vi "Auto_Routine_DepositHighBackup.vi"   [LabVIEW 2020]
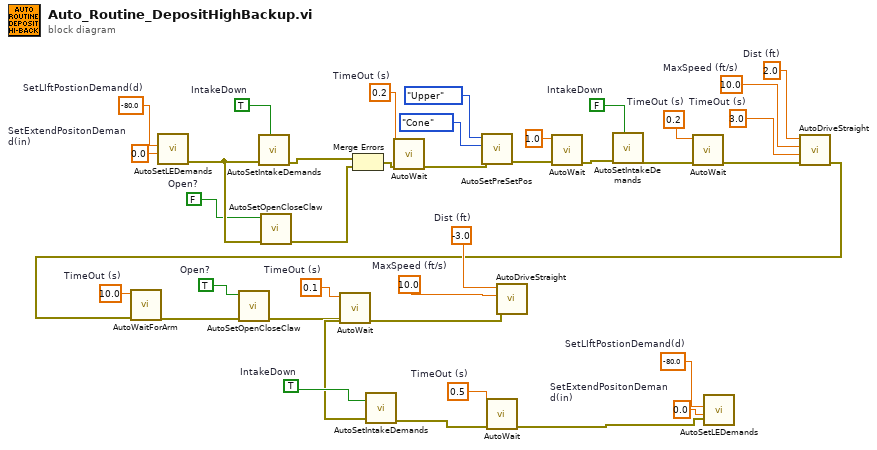
[diagram p0: block diagram]
diagram:
  w30 = 10.0  # MaxSpeed (ft/s)
  w26 = 3.0  # TimeOut (s)
  w25 = 10.0  # MaxSpeed (ft/s)
  w24 = 2.0  # Dist (ft)
  w23 = -80.0  # SetLIftPostionDemand(d)
  w22 = 0.0  # SetExtendPositonDemand(in)
  w21 = 0.5  # TimeOut (s)
  w20 = TRUE  # IntakeDown
  w18 = -3.0  # Dist (ft)
  w17 = 0.1  # TimeOut (s)
  w15 = TRUE  # Open?
  w13 = 0.2  # TimeOut (s)
  w12 = 10.0  # TimeOut (s)
  w7 = FALSE  # IntakeDown
  w5 = 0.2  # TimeOut (s)
  w4 = -80.0  # SetLIftPostionDemand(d)
  w3 = 0.0  # SetExtendPositonDemand(in)
  w2 = FALSE  # Open?
  w1 = TRUE  # IntakeDown
  n1 = call "AutoSetLEDemands.vi"("SetExtendPositonDemand(in)"=w3, "SetLIftPostionDemand(d)"=w4) -> ("error out"=w9:errorcluster)  [unwired: 9 in]
  n2 = call "AutoSetIntakeDemands.vi"("IntakeDown"=w1, "error in (no error)"=w9) -> ("error out"=w27:errorcluster)  [unwired: 9 in]
  n3 = call "AutoSetOpenCloseClaw.vi"("error in (no error)"=w9, "Open?"=w2) -> ("error out"=w28:errorcluster)  [unwired: 9 in]
  n4 = Merge Errors(w27, w28) -> (w29:errorcluster)
  n5 = call "AutoWait.vi"("error in (no error)"=w29, "TimeOut (s)"=w5) -> ("error out"=w6:errorcluster)  [unwired: 9 in]
  n6 = call "AutoSetPreSetPos.vi"("error in (no error)"=w6, "Game Piece"=enum16{"Cube", "Cone"}."Cone", "Position"=enum16{"Upper", "Lower", "Middle"}."Upper") -> ("error out"=w33:errorcluster)  [unwired: 8 in]
  n7 = call "AutoWait.vi"("error in (no error)"=w33, "TimeOut (s)"=1.0) -> ("error out"=w34:errorcluster)  [unwired: 9 in]
  n8 = call "AutoSetIntakeDemands.vi"("IntakeDown"=w7, "error in (no error)"=w34) -> ("error out"=w8:errorcluster)  [unwired: 9 in]
  n9 = call "AutoWait.vi"("error in (no error)"=w8, "TimeOut (s)"=w13) -> ("error out"=w10:errorcluster)  [unwired: 9 in]
  n10 = call "AutoDriveStraight.vi"("error in (no error)"=w10, "TimeOut (s)"=w26, "MaxSpeed (ft/s)"=w25, "Dist (ft)"=w24) -> ("error out"=w11:errorcluster)  [unwired: 7 in]
  n11 = call "AutoWaitForArm.vi"("error in (no error)"=w11, "TimeOut (s)"=w12) -> ("error out"=w14:errorcluster)  [unwired: 9 in]
  n12 = call "AutoSetOpenCloseClaw.vi"("error in (no error)"=w14, "Open?"=w15) -> ("error out"=w16:errorcluster)  [unwired: 9 in]
  n13 = call "AutoWait.vi"("error in (no error)"=w16, "TimeOut (s)"=w17) -> ("error out"=w19:errorcluster)  [unwired: 9 in]
  n14 = call "AutoSetIntakeDemands.vi"("IntakeDown"=w20, "error in (no error)"=w19) -> ("error out"=w31:errorcluster)  [unwired: 9 in]
  n15 = call "AutoWait.vi"("error in (no error)"=w31, "TimeOut (s)"=w21) -> ("error out"=w32:errorcluster)  [unwired: 9 in]
  n16 = call "AutoDriveStraight.vi"("error in (no error)"=w19, "MaxSpeed (ft/s)"=w30, "Dist (ft)"=w18) -> ()  [unwired: 8 in, 1 out]
  n17 = call "AutoSetLEDemands.vi"("error in (no error)"=w32, "SetExtendPositonDemand(in)"=w22, "SetLIftPostionDemand(d)"=w23) -> ()  [unwired: 8 in, 1 out]
